vi "Load State Data.vi"(8 "error in (no error)":errorcluster, 11 "ScrollZoomGraphChart in":refnum<class "ScrollZoomGraphChart.lvclass">) -> (0 "error out":errorcluster, 3 "ScrollZoomGraphChart out":refnum<class "ScrollZoomGraphChart.lvclass">)   [LabVIEW 2025, in "ScrollZoomGraphChart.lvclass"]
doc: "The <b>Load State Data VI</b> is a dynamic dispatch VI that must be overwritten in every QControl Class that uses the State Data. If used it must <b>Call Parent Method</b>. This recursively loads the Data Value Reference to the data space for the QControl Class up the inheritance hierarchy that uses the Data Value Reference.\n<b> </b> <b> </b>\n©2016 Q Software Innovations, LLC (QSI)\nwritten by Quentin Alldredge\nproduced in LabVIEW 2015\n\nsupport@qsoftwareinnovations.com\nwww.qsoftwareinnovations.com\n\nAll rights reserved.\n\nRedistribution and use in source and binary forms, with or without modification, are permitted provided that the following conditions are met:\n\n * Redistributions of source code must retain the above copyright notice, this list of conditions and the following disclaimer.\n * Redistributions in binary form must reproduce the above copyright notice, this list of conditions and the following disclaimer in the documentation and/or other materials provided with the distribution.\n * Neither the name of Q Software Innovations, LLC. nor the names of its contributors may be used to endorse or promote products derived from this software without specific prior written permission.\n\nTHIS SOFTWARE IS PROVIDED BY THE COPYRIGHT HOLDERS AND CONTRIBUTORS \"AS IS\" AND ANY EXPRESS OR IMPLIED WARRANTIES, INCLUDING, BUT NOT LIMITED TO, THE IMPLIED WARRANTIES OF MERCHANTABILITY AND FITNESS FOR A PARTICULAR PURPOSE ARE DISCLAIMED. IN NO EVENT SHALL THE COPYRIGHT OWNER OR CONTRIBUTORS BE LIABLE FOR ANY DIRECT, INDIRECT, INCIDENTAL, SPECIAL, EXEMPLARY, OR CONSEQUENTIAL DAMAGES (INCLUDING, BUT NOT LIMITED TO, PROCUREMENT OF SUBSTITUTE GOODS OR SERVICES; LOSS OF USE, DATA, OR PROFITS; OR BUSINESS INTERRUPTION) HOWEVER CAUSED AND ON ANY THEORY OF LIABILITY, WHETHER IN CONTRACT, STRICT LIABILITY, OR TORT (INCLUDING NEGLIGENCE OR OTHERWISE) ARISING IN ANY WAY OUT OF THE USE OF THIS SOFTWARE, EVEN IF ADVISED OF THE POSSIBILITY OF SUCH DAMAGE."
uses:
  ScrollZoomGraphChart.lvclass
  State Data.ctl
  ScrollZoomGraphChart.lvclass/ScrollZoomGraphChart.ctl
  <vilib>/QSI/QControls/QControl Classes/GraphChart/GraphChart.lvclass
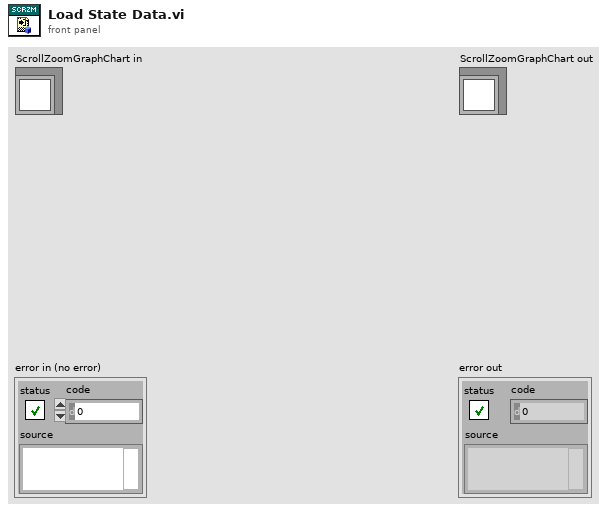
[diagram p1: front panel]
types:
  T1 = typedef "ScrollZoomGraphChart.lvclass/State Data.ctl" = cluster{"X Scales":refnum<vi>[], "Y Scales":refnum<vi>[], "Owning VI":refnum<vi>}
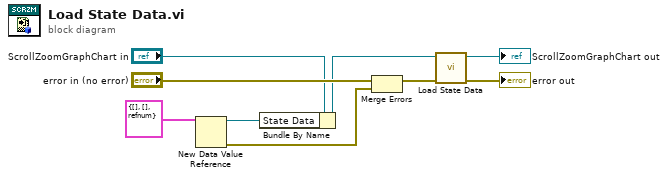
[diagram p0: block diagram]
diagram:
  n1 = New Data Value Reference(data value=T1 {"X Scales"=[], "Y Scales"=[], "Owning VI"=refnum} ("State Data")) -> (data value reference=w4:refnum<data-value>, error out=w2:errorcluster)  [unwired: 1 in]
  n2 = Bundle By Name(cluster="ScrollZoomGraphChart in", "State Data"=w4) -> (w5:refnum<class "ScrollZoomGraphChart.lvclass">)
  n3 = Merge Errors("error in (no error)", w2) -> (w3:errorcluster)
  n4 = call-parent "Load State Data.vi"("error in (no error)"=w3, "Control in"=w5) -> ("error out"=→"error out":errorcluster, "Control out"=→"ScrollZoomGraphChart out":refnum<class "ScrollZoomGraphChart.lvclass">)  [unwired: 8 in]
